vi "SigleDotAdjustment.vi"(9 "adjutFactor":T1 {"旋转参数" format="%0.2f"}, 10 "y":dbl, 11 "x":dbl) -> (2 "y":dbl, 3 "x":dbl)   [LabVIEW 2011]
uses:
  <vilib>/Analysis/coordinate.llb/2D Cartesian Coordinate Shift (Scalar).vi
  <vilib>/Analysis/coordinate.llb/2D Cartesian Coordinate Rotation (Scalar).vi
  <vilib>/Analysis/NI_AALPro.lvlib
panel:
  out "y out":dbl caption="y输出"
  out "x out":dbl caption="x输出"
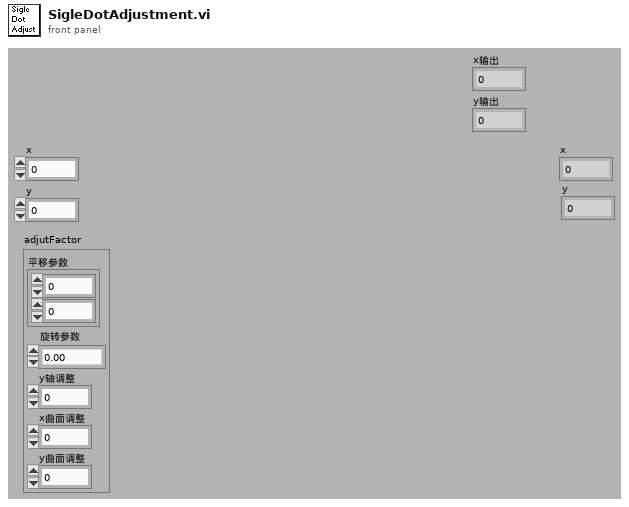
[diagram p1: front panel]
types:
  T1 = cluster{"平移参数":cluster{dbl, dbl}, "旋转参数":dbl, "y轴调整":dbl, "x曲面调整":dbl, "y曲面调整":dbl}
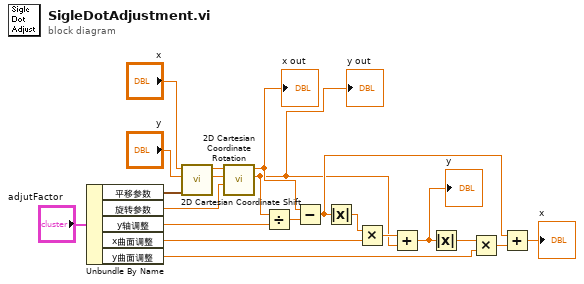
[diagram p0: block diagram]
diagram:
  n1 = Unbundle By Name("adjutFactor") -> ("平移参数"=w19:cluster{dbl, dbl}, "旋转参数"=w14:dbl, "y轴调整"=w13:dbl, "x曲面调整"=w10:dbl, "y曲面调整"=w9:dbl)
  n2 = call-poly <vilib>:"2D Cartesian Coordinate Shift.vi"("shift"=w19, "y"="y", "x"="x") -> ("y out"=w15:dbl, "x out"=w16:dbl)  [unwired: 7 out]
  n3 = call-poly <vilib>:"2D Cartesian Coordinate Rotation.vi"("theta"=w14, "y"=w15, "x"=w16) -> ("y out"=w1:dbl, "x out"=w2:dbl)  [unwired: 7 out]
  "x out" <- w2
  "y out" <- w1
  n4 = Divide(x=w1, y=w13) -> (x/y=w12:dbl)
  n5 = Subtract(x=w2, y=w12) -> (x-y=w4:dbl)
  n6 = Absolute Value(x=w4) -> (abs(x)=w11:dbl)
  n7 = Multiply(x=w11, y=w10) -> (x*y=w7:dbl)
  n8 = Add(x=w7, y=w1) -> (x+y=w5:dbl)
  "y" <- w5
  n9 = Absolute Value(x=w5) -> (abs(x)=w6:dbl)
  n10 = Multiply(x=w6, y=w9) -> (x*y=w8:dbl)
  n11 = Add(x=w4, y=w8) -> (x+y=→"x":dbl)
